vi "UEvent_ON_OFF_POWER_SOURCE.vi"(6 "USB":tag, 7 "Power ON/OFF DUT":enum16{"Power ON DUT", "Power OFF DUT"}(ring), 9 "Value":T1, 10 "Vout  - Vbat profile":enum16{"3.8VDC", "2.9VDC", "3.7VDC", "4.0VDC"}(ring), 11 "Refnum in":refnum<k21>) -> (1 "Battery_Voltage":dbl, 2 "DUT_Voltage":dbl, 3 "Refnum out":refnum<k21>)   [LabVIEW 2015]
uses:
  Range_Shunt_selector.ctl
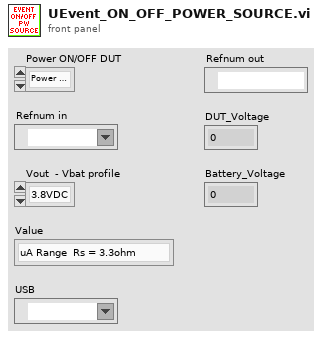
[diagram p1: front panel]
types:
  T1 = typedef "Range_Shunt_selector.ctl" = enum16{"uA Range  Rs = 3.3ohm", "mA Range Rs = 3.3Ohm", "mA Range Rs = 1Ohm", "mA Range Rs = 1Ohm - X2"}
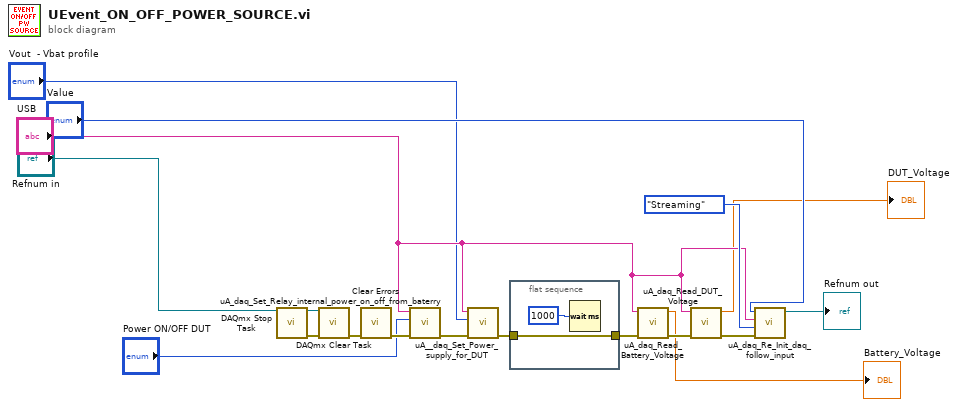
[diagram p0: block diagram]
diagram:
  n1 = call <vilib>:"DAQmx Stop Task.vi"("task/channels in"="Refnum in") -> ("task out"=w4:refnum<k21>, "error out"=w1:errorcluster)  [unwired: 13 in]
  n2 = call <vilib>:"DAQmx Clear Task.vi"("task in"=w4, "error in"=w1) -> ("error out"=w2:errorcluster)  [unwired: 13 in]
  n3 = call <vilib>:"Clear Errors.vi"("error in (no error)"=w2) -> ("error out"=w8:errorcluster)  [unwired: 5 in, 1 out]
  n4 = call "uA_daq_Set_Relay_internal_power_on_off_from_baterry.vi"("error in"=w8, "Power ON/OFF DUT"="Power ON/OFF DUT", "USB DAQ"="USB") -> ("error out"=w11:errorcluster)  [unwired: 8 in]
  n5 = call "uA__daq_Set_Power_supply_for_DUT.vi"("error in"=w11, "DUT Voltage Selector"="Vout  - Vbat profile", "USB DAQ"="USB") -> ("error out"=w12:errorcluster)  [unwired: 8 in]
  n6 = flat-sequence {
    tunnel: w12 -> [w20]
    tunnel: [w20] -> w13
    frame #0 {
      n7 = Wait (ms)(milliseconds to wait=u32 1000) -> ()  [unwired: 1 out]
    }
  }
  n8 = call "uA_daq_Read_Battery_Voltage.vi"("error in"=w13, "USB DAQ"="USB") -> ("error out"=w9:errorcluster, "Battery_Voltage"=→"Battery_Voltage":dbl)  [unwired: 8 in]
  n9 = call "uA_daq_Read_DUT_Voltage.vi"("error in"=w9, "USB DAQ"="USB") -> ("error out"=w18:errorcluster, "DUT_Voltage"=→"DUT_Voltage":dbl)  [unwired: 8 in]
  n10 = call "uA_daq_Re_Init_daq_follow_input.vi"("error in (no error)"=w18, "Acquire Mode"=enum16{"Streaming", "Read All", "Stop"}."Streaming", "USB"="USB", "Range_shunt"="Value") -> ("Refnum out"=→"Refnum out":refnum<k21>)  [unwired: 6 in, 1 out]
